vi "Read Data From Gif File.vi"(0 "Gif File Path":path, 3 "error in (no error)":errorcluster caption="错误输入（无错误）") -> (7 "Gif Image 输出":refnum<class "Gif Image.lvclass"> caption="DNL_LabVIEW Object out", 10 "error out":errorcluster caption="错误输出")   [LabVIEW 2012, in "Picture Box Tools.lvlib" / "Gif Image.lvclass"]
uses:
  Gif Image.lvclass
  Gif Image.lvclass/Gif Image.ctl
panel:
  in  "Gif Image 输入":refnum<class "Gif Image.lvclass"> caption="DNL_LabVIEW Object in"
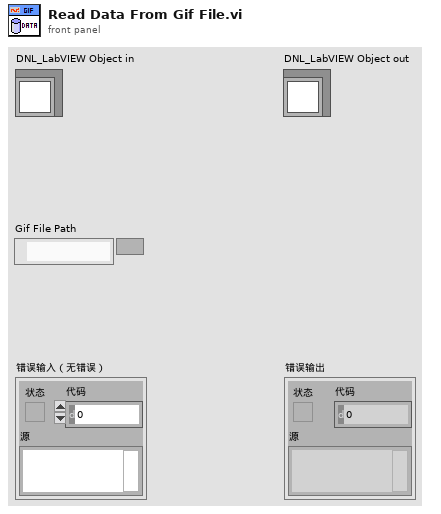
[diagram p1: front panel]
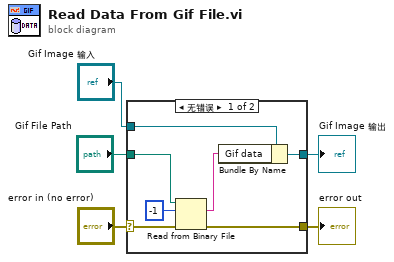
[diagram p0: block diagram]
diagram:
  n1 = case shown="无错误" "error in (no error)" {
    selector: "error in (no error)" -> [w10 w14]
    tunnel: [w9 w14] -> w4
    tunnel: [w6 w13] -> w2
    tunnel: "Gif Image 输入" -> [w8 w13]
    tunnel: "Gif File Path" -> [w11 _]
    frame No Error {
      n2 = Read from Binary File(8:w10, 10:-1 ("总数(1)"), 11:w11) -> (0:w9:errorcluster, 2:w7:string)  [unwired: 3 in, 2 out]
      n3 = Bundle By Name(cluster=w8, "Gif data"=w7) -> (w6:refnum<class "Gif Image.lvclass">)
    }
    frame Error {
    }
  }
  "error out" <- w4
  "Gif Image 输出" <- w2
